vi "Hipot_RST.vi"(8 "Error In":errorcluster, 10 "PORT":string, 11 "Limit":string="AC~5~0.1~0.0") -> (0 "Error Out":errorcluster, 2 "Result":bool, 3 "Data":string)   [LabVIEW 2013]
uses:
  MainProgram/Control/Buffer.vi
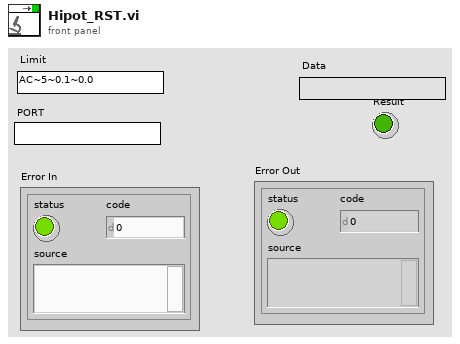
[diagram p1: front panel]
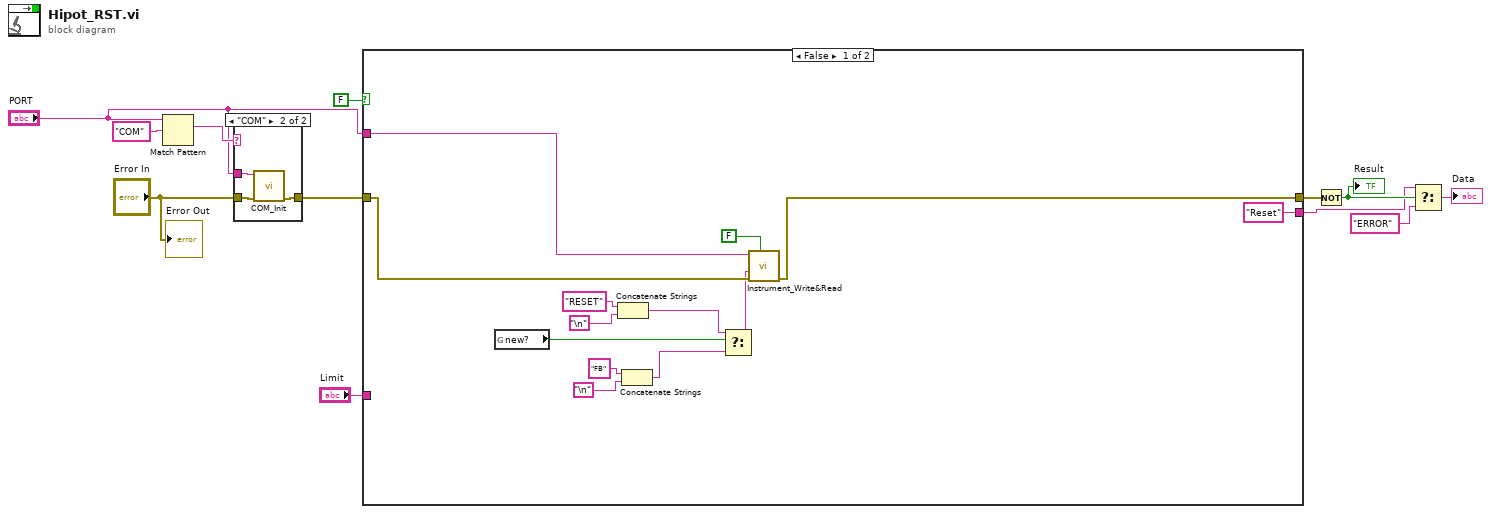
[diagram p0: block diagram]
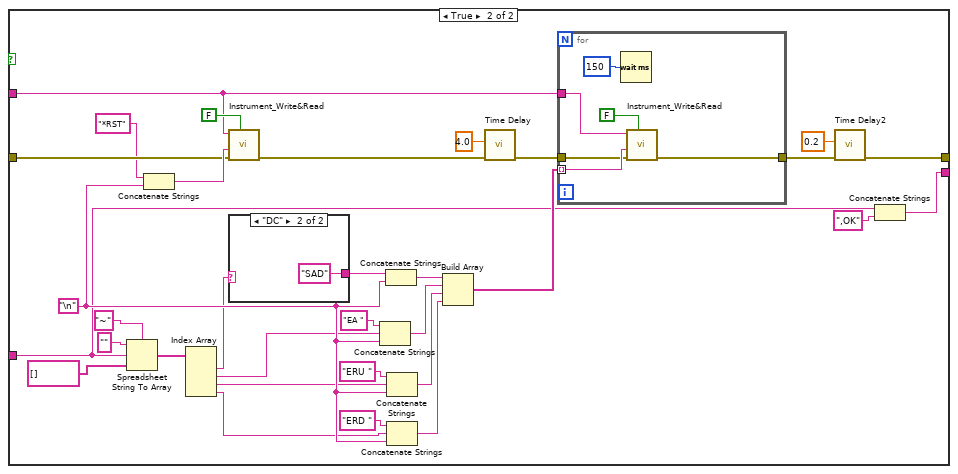
[diagram p3: hidden frame]
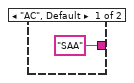
[diagram p4: hidden frame]
diagram:
  n1 = Match Pattern(string="PORT", regular expression="COM") -> (match substring=w5:string)  [unwired: 1 in, 3 out]
  n2 = case shown="\"COM\"" w5 {
    tunnel: "PORT" -> [_ w16]
    tunnel: "Error In" -> [w13 w15]
    tunnel: [w13 w14] -> w3
    frame Default {
    }
    frame "COM" {
      n3 = call "COM_Init.vi"("error in (no error)"=w15, "VISA Refnum in"=w16) -> ("error out"=w14:errorcluster)  [unwired: 8 in, 1 out]
    }
  }
  n4 = case shown="False" FALSE {
    tunnel: [w25 w51] -> w9
    tunnel: "Limit" -> [_ w37]
    tunnel: w3 -> [w26 w33]
    tunnel: ["Reset" w36] -> w7
    tunnel: "PORT" -> [w27 w31]
    frame False {
      n5 = global read "Buffer.vi" "new?"() -> (w22:bool)
      n6 = Concatenate Strings("RESET" ("Characters to Write"), "\n") -> (w21:string)
      n7 = Concatenate Strings("FB" ("Characters to Write"), "\n") -> (w17:string)
      n8 = Select(t=w21, s=w22, f=w17) -> (s? t:f=w20:string)
      n9 = call "Instrument_Write&Read.vi"("Read?"=FALSE, "Error In"=w26, "CMD"=w20, "PORT"=w27) -> ("Error Out"=w25:errorcluster)  [unwired: 6 in, 1 out]
    }
    frame True {
      w48 = "\n"
      n10 = Spreadsheet String To Array(delimiter (Tab)="~", format string="", spreadsheet string=w37, array type (2D Dbl)=string[] []) -> (array=w43:string[])
      n11 = Concatenate Strings("*RST" ("Characters to Write"), w48) -> (w34:string)
      n12 = Index Array(array=w43) -> (element #1=w39:string, element #2=w42:string, element #3=w41:string, element #4=w40:string)  [unwired: 4 in]
      n13 = call "Instrument_Write&Read.vi"("Read?"=FALSE, "Error In"=w33, "CMD"=w34, "PORT"=w31) -> ("Error Out"=w32:errorcluster)  [unwired: 6 in, 1 out]
      n14 = case shown="\"DC\"" w39 {
        tunnel: ["SAA" ("写入缓冲区") "SAD" ("写入缓冲区")] -> w49
        frame "AC", Default {
        }
        frame "DC" {
        }
      }
      n15 = Concatenate Strings("EA " ("字符串"), w42, w48) -> (w57:string)
      n16 = Concatenate Strings(w49, w48) -> (w47:string)
      n17 = Concatenate Strings("ERU " ("字符串"), w41, w48) -> (w56:string)
      n18 = Concatenate Strings("ERD " ("字符串"), w40, w48) -> (w55:string)
      n19 = Build Array(w47, w57, w56, w55) -> (w54:string[])
      n20 = call "Time Delay"("error in (no error)"=w32, "Delay Time (s)"=4.0) -> ("error out"=w53:errorcluster)  [unwired: 9 in]
      n21 = for {
        tunnel: w54 -> [w66] mode=indexing
        tunnel: w53 -> [w65]
        tunnel: [w64] -> w50
        tunnel: w31 -> [w67]
        n22 = Wait (ms)(milliseconds to wait=u32 150) -> ()  [unwired: 1 out]
        n23 = call "Instrument_Write&Read.vi"("Read?"=FALSE, "Error In"=w65, "CMD"=w66, "PORT"=w67) -> ("Error Out"=w64:errorcluster)  [unwired: 6 in, 1 out]
      }
      n24 = call "Time Delay2"("error in (no error)"=w50, "Delay Time (s)"=0.2) -> ("error out"=w51:errorcluster)  [unwired: 9 in]
      n25 = Concatenate Strings(w37, ",OK") -> (w36:string)
    }
  }
  n26 = Not(x=w9) -> (.not. x?=w10:bool)
  "Result" <- w10
  n27 = Select(t=w7, s=w10, f="ERROR") -> (s? t:f=→"Data":string)
  "Error Out" <- "Error In"
